vi "Create_Object.vi"(8 "error in (no error)":errorcluster, 9 "Terminal Map in":map{string, T1}(c390), 10 "owner refnum":variant, 11 "String Control in":refnum<class "String Control.lvclass">) -> (0 "error out":errorcluster, 1 "Terminal Map Out":map{string, T1}(c390), 3 "String Control out":refnum<class "String Control.lvclass">)   [LabVIEW 2025, in "String Control.lvclass"]
uses:
  String Control.lvclass
  Controls/Terminal.ctl
  Node.lvclass/Node.ctl
  Control.lvclass
  String Control.lvclass/String Control.ctl
  Node.lvclass
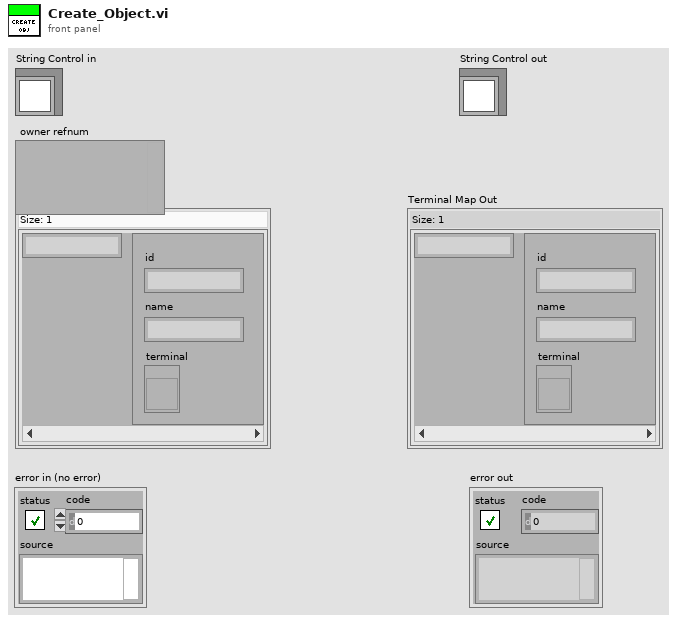
[diagram p1: front panel]
types:
  T1 = typedef "Terminal.ctl" = cluster{"id":string, "name":string, "terminal":refnum<vi>}
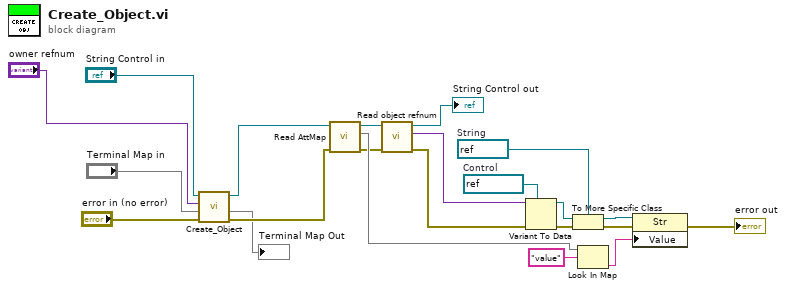
[diagram p0: block diagram]
diagram:
  w17 = refnum<vi> refnum  # String
  w18 = refnum<vi> refnum  # Control
  n1 = call-parent "Create_Object.vi"("error in (no error)"="error in (no error)", "Terminal Map in"="Terminal Map in", "owner refnum"="owner refnum", "Control in"="String Control in") -> ("error out"=w10:errorcluster, "Terminal Map Out"=→"Terminal Map Out":map{string, T1}, "Control out"=w11:refnum<class "String Control.lvclass">)  [unwired: 5 in]
  n2 = call "Read AttMap.vi"("error in (no error)"=w10, "Node in"=w11) -> ("error out"=w8:errorcluster, "AttMap"=w9:map{string, string}, "Node out"=w7:refnum<class "String Control.lvclass">)  [unwired: 7 in]
  n3 = call-dynamic "Read object refnum.vi"("error in (no error)"=w8, "Node in"=w7) -> ("error out"=w3:errorcluster, "object refnum"=w6:variant, "Node out"=→"String Control out":refnum<class "String Control.lvclass">)  [unwired: 7 in]
  n4 = Variant To Data(error in=w3, type=w18, Variant=w6) -> (data=w16:refnum<vi>, error out=w15:errorcluster)
  n5 = To More Specific Class(target class=w17, reference=w16, error in=w15) -> (specific class reference=w19:refnum<vi>, error out=w14:errorcluster)
  n6 = Look In Map(map=w9, key="value" ("valueConst")) -> (value=w12:string)  [unwired: 1 in, 1 out]
  n7 = property class="Str"(reference=w19, error in=w14, "Value"=w12) -> (error out=→"error out":errorcluster)  [unwired: 1 out]
